vi "template.vi"() -> ()   [LabVIEW 2020]
uses:
  <vilib>/Platform/TimedLoop/XDataNode/timing_clust.ctl
  <vilib>/Platform/TimedLoop/XDataNode/nitl_modes.ctl
  <vilib>/Platform/TimedLoop/XDataNode/wakeup.ctl
  <extravilib>/ChannelInstances/Stream-bool/Write With Abort.vi
  <extravilib>/ChannelInstances/Stream-bool/Read With Abort.vi
  <extravilib>/ChannelInstances/Stream-bool/Endpoint.vi
  <extravilib>/ChannelInstances/Stream-bool/EndpointRead.vi
  <extravilib>/ChannelInstances/Stream-bool/Instantiate.vi
  <extravilib>/ChannelInstances/Stream-bool/)Channel.vi
  <resource>/ChannelSupport/_ChannelSupport/WaitIfNeeded.vi
  <vilib>/platform/TimedLoop/XDataNode/XDataNode.xnode
  <vilib>/Platform/TimedLoop/XDataNode/XDNodeRunTimeDep.lvlib
  <extravilib>/ChannelInstances/Stream-bool.lvlib
panel:
  out "Numeric":i32
  out "error out":errorcluster
  out "GPS data out":string
  in  "Stop":bool
  out "Arm System":bool
  in  "Start":bool
  out "Laser 2":bool
  out "Laser 1":bool
  in  "Speed Threshold (km/h)":dbl
  out "Safety System 2":bool[](array[boolean])
  out "Safety System 1":bool[](array[boolean])
  out "GPS":cluster{"Lat":dbl, "Lon":dbl, "Speed":dbl}
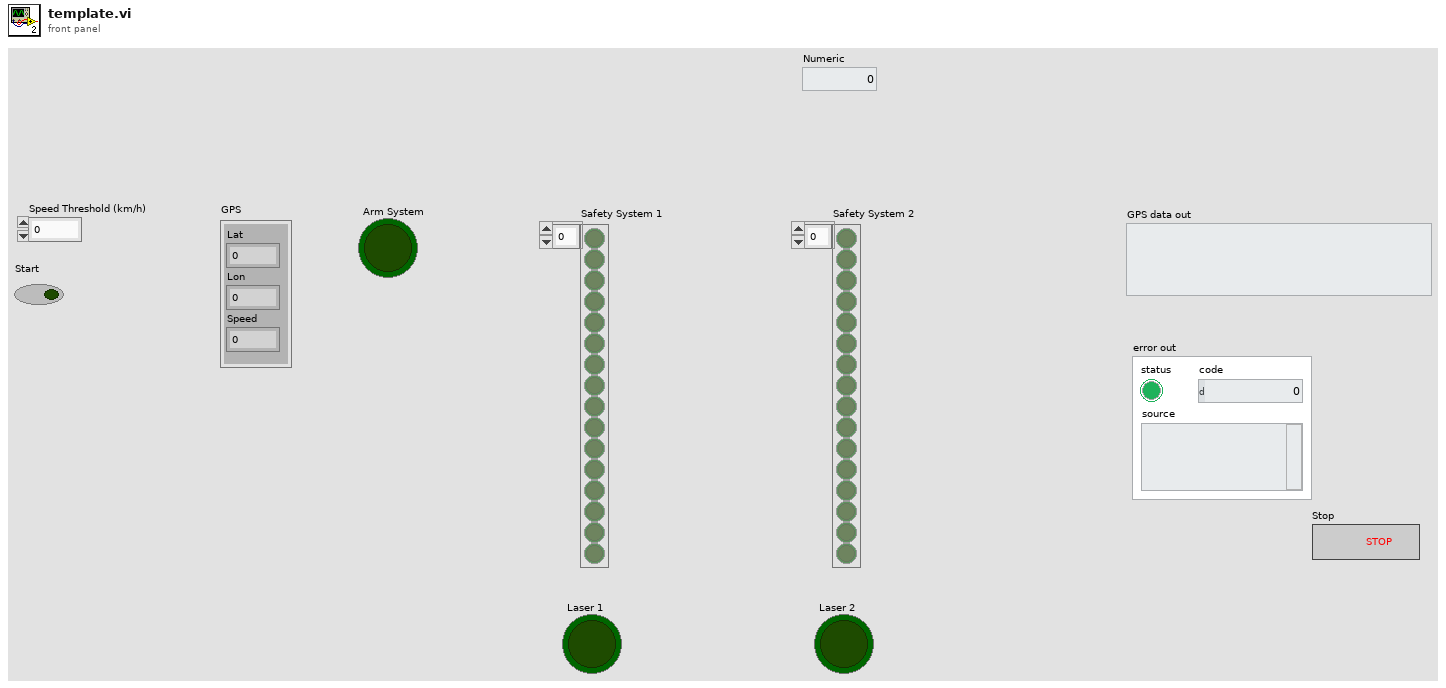
[diagram p1: front panel]
types:
  T1 = enum16{"Standard", "Buffered", "CRLF", "Immediate"}
  T2 = typedef "XDNodeRunTimeDep.lvlib/timing_clust.ctl" = cluster{"Expected End [f-1]":u64, "Actual End [f-1]":u64, "Finished Late? [f-1]":bool, "Expected End [i-1]":u64, "Actual End [i-1]":u64, "Finished Late? [i-1]":bool, "Expected Start [i]":u64, "Actual Start [i]":u64, "Expected Start [f]":u64, "Actual Start [f]":u64, "Source Name":string, "Structure Name":string, "Period":i64, "Deadline":i64, "Offset":i64, "Start":i64, "Priority":i32, "Timeout":i32, "Mode":T3, "Wakeup Reason":T4, "Error":errorcluster, "Source Type":string, "Secondary Source Type":string, "Global End Time":u64, "Global Start Time":u64, "Frame Duration":u64, "Iteration Duration":u64, "Assigned CPU":i32, "I/O Scan Engine Mode":u32}
  T3 = typedef "XDNodeRunTimeDep.lvlib/nitl_modes.ctl" = enum32{"No Change", "Process missed periods, maintain original phase", "Discard missed periods, maintain original phase", "Process missed periods, ignore original phase", "Discard missed periods, ignore original phase"}
  T4 = typedef "XDNodeRunTimeDep.lvlib/wakeup.ctl" = enum32{"Normal", "Aborted", "Asynchronous wakeup", "Timing source error", "Timed loop error", "Timeout"}
  T5 = typedef "Stream-bool.lvlib/)Channel.ctl" = refnum<queue>
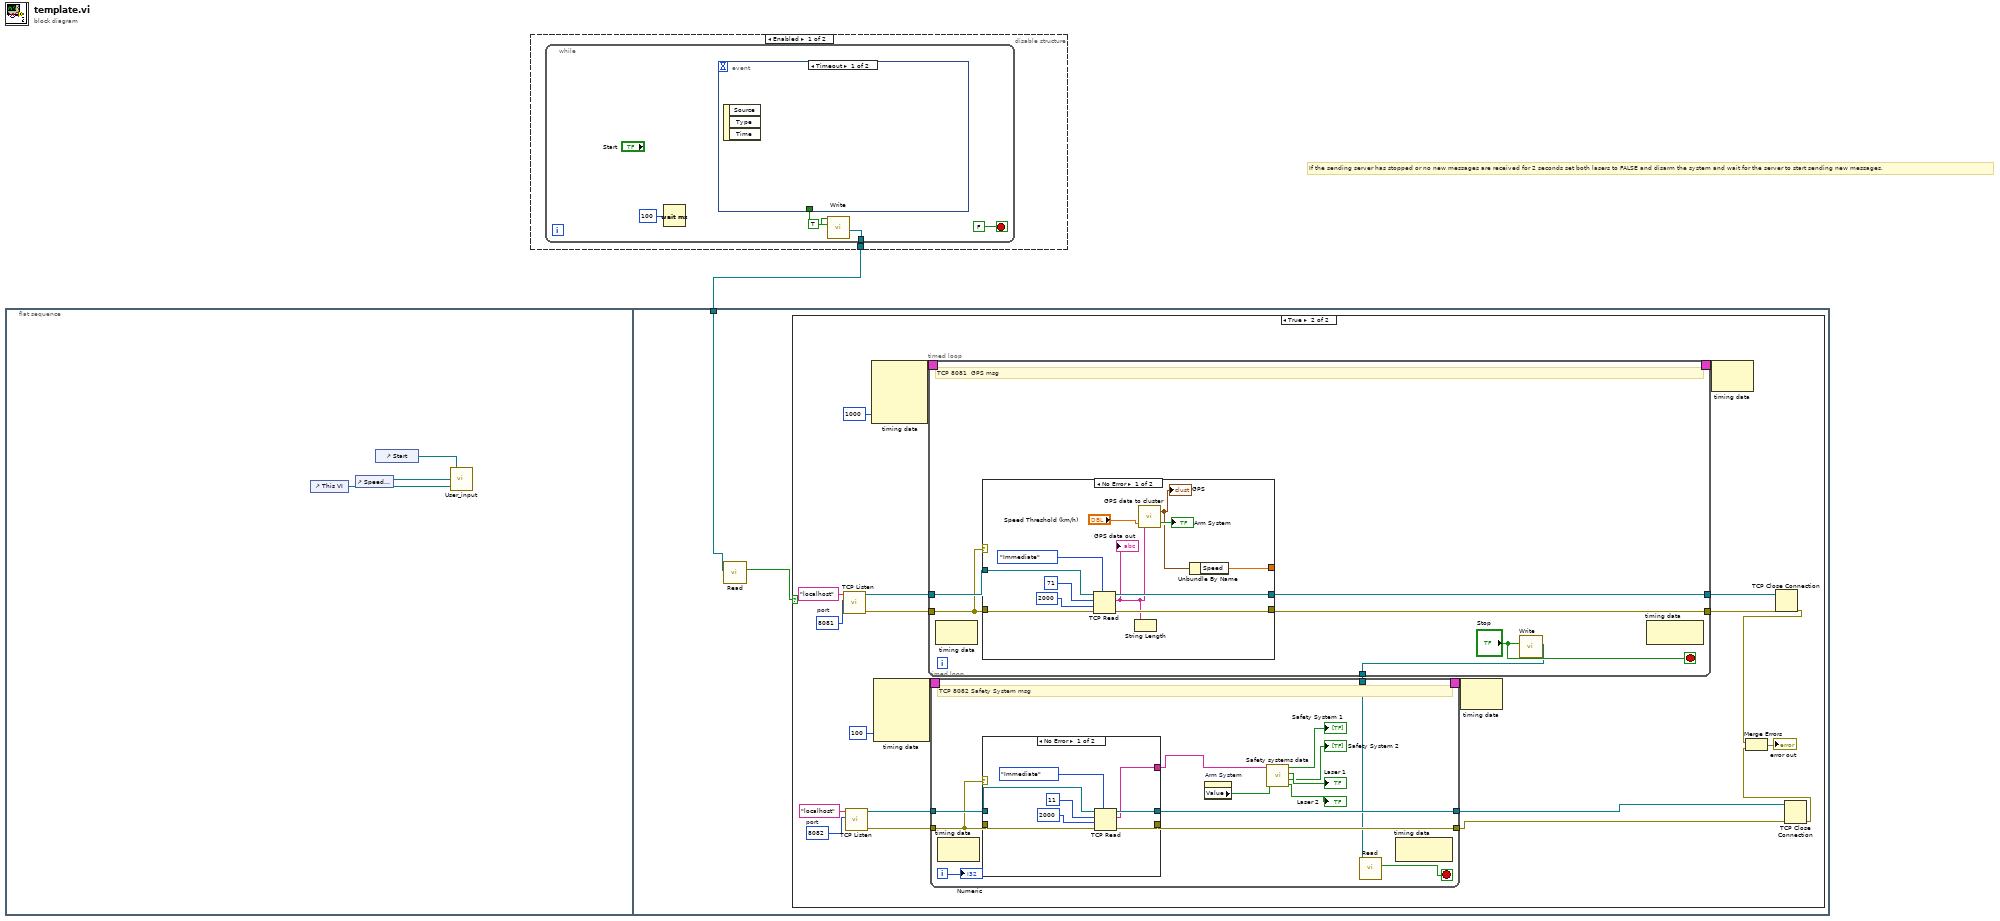
[diagram p0: block diagram]
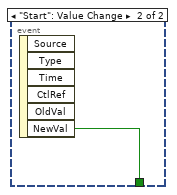
[diagram p2: hidden frame]
diagram:
  # "If the sending server has stopped or no new messages are received for 2 seconds set both lasers to FALSE and disarm the system and wait for the server to start sending new messages."
  n1 = flat-sequence {
    tunnel: w1 -> [w5]
    frame #0 {
      n2 = control-ref of="This VI"() -> (w2:refnum<vi>)
      n3 = control-ref of="Speed Threshold (km/h)"() -> (w3:refnum<vi>)
      n4 = control-ref of="Start"() -> (w4:refnum<vi>)
      n5 = call "User_input.vi"("Main Vi"=w2, "Speed Threshold (km/h) Ref"=w3, "Start Ref"=w4) -> ()  [unwired: 1 in]
    }
    frame #1 {
      n6 = call <extravilib>:"Read.vi"("channel"=w5) -> ("element"=w6:bool)  [unwired: 6 in, 4 out]
      n7 = case shown="True" w6 {
        frame False {
        }
        frame True {
          w18 = u16 8082  # port
          w24 = u16 8081  # port
          n8 = call <vilib>:"TCP Listen.vi"("port"=w24, "service name"="localhost") -> ("error out"=w22:errorcluster, "connection ID"=w15:refnum<k5>)  [unwired: 5 in, 3 out]
          n9 = call <vilib>:"TCP Listen.vi"("port"=w18, "service name"="localhost") -> ("error out"=w20:errorcluster, "connection ID"=w21:refnum<k5>)  [unwired: 5 in, 3 out]
          n10 = node-c288(i64 1000 ("Period")) -> (w28:T2)  [unwired: 3 in]
          n11 = node-c288(i64 100 ("Period")) -> (w26:T2)  [unwired: 3 in]
          n12 = timed-loop {
            tunnel: w22 -> [w60]
            tunnel: w15 -> [w63]
            tunnel: [w62] -> w14
            tunnel: [w61] -> w13
            timing: w28 -> [_]
            timing-out: [_] -> w27
            tunnel: [w58] -> w7
            stop <- "Stop" stop-if-true
            # "TCP 8081  GPS msg"
            n13 = node-c288() -> ()  [unwired: 1 in, 1 out]
            n14 = case shown="No Error" w60 {
              tunnel: w60 -> [w72 w77]
              tunnel: w63 -> [w71 w76]
              tunnel: [w70 w77] -> w62
              tunnel: [w69 w76] -> w61
              tunnel: [w65 _] -> _
              frame No Error {
                n15 = TCP Read(connection ID=w71, bytes to read=71, error in (no error)=w72, 7:T1."Immediate" ("mode (standard)"), 9:2000 ("timeout ms (25000)")) -> (connection ID out=w69:refnum<k5>, data out=w64:string, error out=w70:errorcluster)
                "GPS data out" <- w64
                n16 = String Length(string=w64) -> ()  [unwired: 1 out]
                n17 = call "GPS data to cluster.vi"("Speed Threshold (km/h)"="Speed Threshold (km/h)", "Gps raw data in"=w64) -> ("Arm System?"=→"Arm System":bool, "GPS Cluster"=w66:cluster{"Lat":dbl, "Lon":dbl, "Speed":dbl})
                "GPS" <- w66
                n18 = Unbundle By Name(w66) -> ("Speed"=w65:dbl)
              }
              frame Error {
              }
            }
            n19 = call <extravilib>:"Write.vi"("element"="Stop") -> ("channel"=w58:T5)  [unwired: 8 in, 2 out]
            n20 = node-c288() -> ()  [unwired: 1 in, 1 out]
          }
          n21 = timed-loop {
            tunnel: w20 -> [w32]
            tunnel: w21 -> [w41]
            tunnel: [w40] -> w12
            tunnel: [w39] -> w11
            timing: w26 -> [_]
            timing-out: [_] -> w25
            tunnel: w7 -> [w30]
            i -> [w29]
            stop <- w31 stop-if-true
            # "TCP 8082 Safety System msg"
            n22 = node-c288() -> ()  [unwired: 1 in, 1 out]
            n23 = case shown="No Error" w32 {
              tunnel: w32 -> [w46 w51]
              tunnel: w41 -> [w45 w50]
              tunnel: [w44 w51] -> w40
              tunnel: [w43 w50] -> w39
              tunnel: [w42 _] -> w38
              frame No Error {
                n24 = TCP Read(connection ID=w45, bytes to read=11, error in (no error)=w46, 7:T1."Immediate" ("mode (standard)"), 9:2000 ("timeout ms (25000)")) -> (connection ID out=w43:refnum<k5>, data out=w42:string, error out=w44:errorcluster)
              }
              frame Error {
              }
            }
            n25 = property on="Arm System" class="Bool (strict)"() -> ("Value"=w33:bool)  [unwired: 2 in, 2 out]
            n26 = call "Safety systems data.vi"("Arm System Status"=w33, "safety system raw data"=w38) -> ("Laser 2"=→"Laser 2":bool, "Safety System 2"=→"Safety System 2":bool[], "Laser 1"=→"Laser 1":bool, "Safety System 1"=→"Safety System 1":bool[])  [unwired: 3 in]
            n27 = call <extravilib>:"Read.vi"("channel"=w30) -> ("element"=w31:bool)  [unwired: 6 in, 4 out]
            n28 = node-c288() -> ()  [unwired: 1 in, 1 out]
            "Numeric" <- w29
          }
          n29 = node-c288(w25) -> ()  [unwired: 1 out]
          n30 = node-c288(w27) -> ()  [unwired: 1 out]
          n31 = TCP Close Connection(connection ID=w13, error in (no error)=w14) -> (error out=w9:errorcluster)  [unwired: 1 in, 1 out]
          n32 = TCP Close Connection(connection ID=w11, error in (no error)=w12) -> (error out=w8:errorcluster)  [unwired: 1 in, 1 out]
          n33 = Merge Errors(w9, w8) -> (→"error out":errorcluster)
        }
      }
    }
  }
  n34 = disable-structure shown="Enabled" {
    disable-tunnel: [w84 _] -> w1
    frame Enabled {
      n35 = while {
        tunnel: [w85] -> w84
        stop <- FALSE stop-if-true
        n36 = Wait (ms)(milliseconds to wait=u32 100) -> ()  [unwired: 1 out]
        n37 = event shown="[0] Timeout" {
          selector: _ -> [_ _]
          dyn-events: _ -> [_ _]
          timeout: _ -> [_ _]
          tunnel: [_ w90] -> w87
          event Timeout {
            n38 = event-data() -> ()  [unwired: 1 in, 3 out]
          }
          event "Start": Value Change {
            n39 = event-data() -> ("NewVal"=w90:bool)  [unwired: 1 in, 5 out]
          }
        }
        n40 = call <extravilib>:"Write.vi"("element"=w87, "element valid? (T)"=TRUE) -> ("channel"=w85:T5)  [unwired: 7 in, 2 out]
      }
    }
    frame Disabled {
    }
  }
